vi "G#Object_GetAllObjects.vi"(1 "full class name (\"\")":string, 2 "only refs (F)":bool, 5 "error in (no error)":errorcluster) -> (10 "all objects":T1[](array[typedef]), 12 "all refs":refnum<class "G#Object.lvclass">[](array[class]), 15 "class information":T3[](array[typedef]), 19 "error out":errorcluster)   [LabVIEW 2017, in "G#Object.lvclass"]
doc: "Returns all objects of the specified class. If \"full class name\" is empty, all objects of all classes will be returned."
uses:
  G#Object.lvclass
  G#Object_ClassInfoType.ctl
  G#Object_ObjectInfoType.ctl
  G#Object_CreateMethod.ctl
  G#Object.lvclass/G#Object.ctl
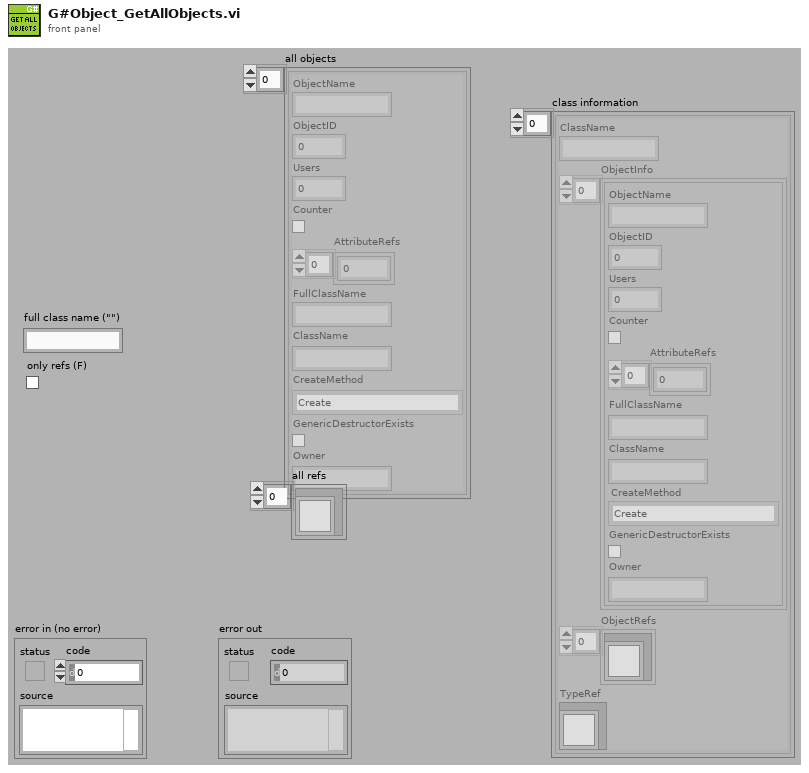
[diagram p1: front panel]
types:
  T1 = typedef "G#Object.lvclass/G#Object_ObjectInfoType.ctl" = cluster{"ObjectName":string, "ObjectID":u32, "Users":i32, "Counter":bool, "AttributeRefs":u32[], "FullClassName":string, "ClassName":string, "CreateMethod":T2, "GenericDestructorExists":bool, "Owner":string}
  T2 = typedef "G#Object.lvclass/G#Object_CreateMethod.ctl" = enum16{"Create", "Create or look up existing", "Look up existing"}
  T3 = typedef "G#Object.lvclass/G#Object_ClassInfoType.ctl" = cluster{"ClassName":string, "ObjectInfo":T1[], "ObjectRefs":refnum<class "G#Object.lvclass">[], "TypeRef":refnum<class "G#Object.lvclass">}
  T4 = cluster{"full class name (\"\")":string, "Ref":refnum<class "G#Object.lvclass">}
  T5 = cluster{"full class name (\"\")":string, "Ref":refnum<class "G#Object.lvclass">}[]
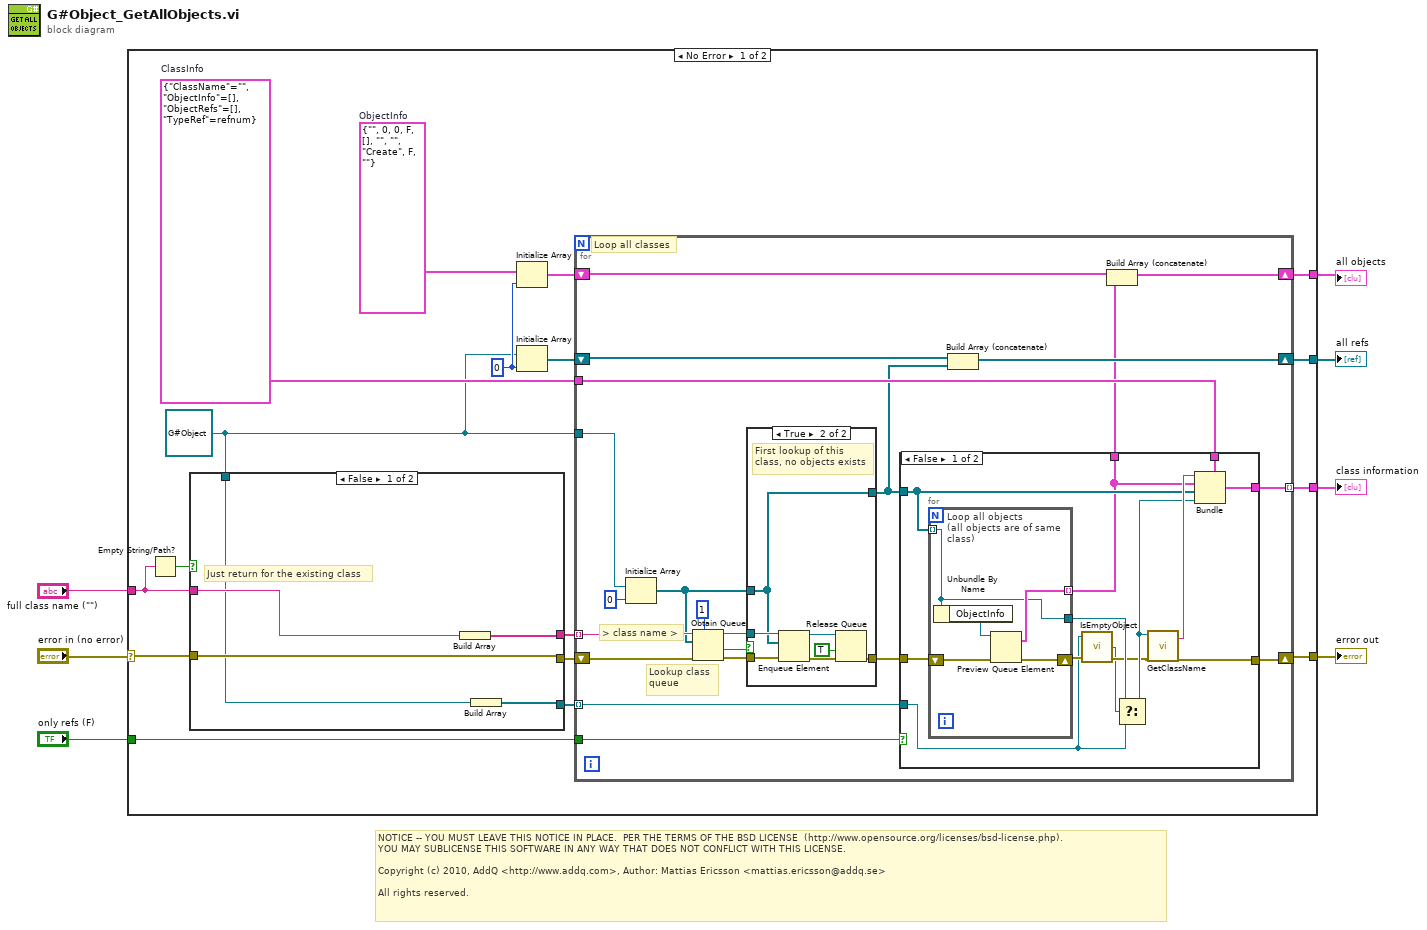
[diagram p0: block diagram]
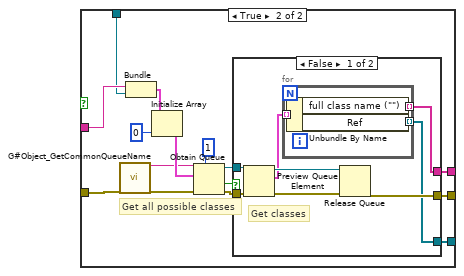
[diagram p2: hidden frame]
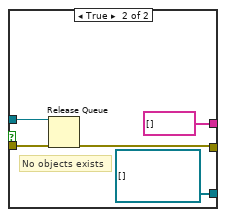
[diagram p3: hidden frame]
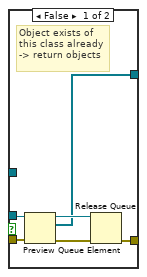
[diagram p5: hidden frame]
diagram:
  # "NOTICE -- YOU MUST LEAVE THIS NOTICE IN PLACE.  PER THE TERMS OF THE BSD LICENSE  (http://www.opensource.org/licenses/bsd-license.php).\nYOU MAY SUBLICENSE THIS SOFTWARE IN ANY WAY THAT DOES NOT CONFLICT WITH THIS LICENSE.\n\nCopyright (c) 2010, AddQ <http://www.addq.com>, Author: Mattias Ericsson <mattias.ericsson@addq.se>\n\nAll rights reserved."
  n1 = case shown="No Error" "error in (no error)" {
    selector: "error in (no error)" -> [w20 w114]
    tunnel: [w14 w114] -> w6
    tunnel: [w18 _] -> w5
    tunnel: [w19 _] -> w4
    tunnel: [w15 _] -> w3
    tunnel: "only refs (F)" -> [w13 _]
    tunnel: "full class name (\"\")" -> [w11 _]
    frame No Error {
      w9 = refnum<class "G#Object.lvclass"> refnum ("Ref")
      w10 = T1 {"ObjectName"="", "ObjectID"=0, "Users"=0, "Counter"=FALSE, "AttributeRefs"=[], "FullClassName"="", "ClassName"="", "CreateMethod"=enum."Create", "GenericDestructorExists"=FALSE, "Owner"=""}  # ObjectInfo
      w21 = T3 {"ClassName"="", "ObjectInfo"=[], "ObjectRefs"=[], "TypeRef"=refnum}  # ClassInfo
      w16 = 0 ("dimension size")
      n2 = Empty String/Path?(string/path=w11) -> (empty?=w12:bool)
      n3 = case shown="False" w12 {
        tunnel: [w28 w38] -> w23
        tunnel: [w29 w37] -> w22
        tunnel: w20 -> [w29 w32]
        tunnel: w11 -> [w27 w35]
        tunnel: w9 -> [w26 w33]
        tunnel: [w25 w34] -> w8
        frame False {
          # "Just return for the existing class"
          n4 = Build Array(w27) -> (w28:string[])
          n5 = Build Array(w26) -> (w25:refnum<class "G#Object.lvclass">[])
        }
        frame True {
          # "Get all possible classes"
          n6 = call "G#Object_GetCommonQueueName.vi"("error in (no error)"=w32) -> ("queue name"=w30:string, "error out"=w31:errorcluster)  [unwired: 17 in]
          n7 = Bundle("full class name (\"\")"=w35, "Ref"=w33) -> (w36:T4)  [unwired: 1 in]
          n8 = Initialize Array(w36, 0 ("dimension size")) -> (w39:T5)
          n9 = Obtain Queue(max queue size (-1, unlimited)=1, name (unnamed)=w30, element data type=w39, error in (no error)=w31) -> (queue out=w42:refnum<queue>, created new?=w44:bool, error out=w43:errorcluster)  [unwired: 1 in]
          n10 = case shown="False" w44 {
            tunnel: w43 -> [w52 w57]
            tunnel: w42 -> [w51 w58]
            tunnel: [w47 string[] []] -> w38
            tunnel: [w50 w60] -> w37
            tunnel: [w45 refnum<class "G#Object.lvclass">[] []] -> w34
            frame False {
              # "Get classes"
              n11 = Preview Queue Element(queue=w51, error in (no error)=w52) -> (queue out=w48:refnum<queue>, element=w46:T5, error out=w49:errorcluster)  [unwired: 1 in, 1 out]
              n12 = for {
                tunnel: [w55] -> w47 mode=indexing
                tunnel: w46 -> [w54] mode=indexing
                tunnel: [w53] -> w45 mode=indexing
                n13 = Unbundle By Name(w54) -> ("full class name (\"\")"=w55:string, "Ref"=w53:refnum<class "G#Object.lvclass">)
              }
              n14 = Release Queue(queue=w48, error in (no error)=w49) -> (error out=w50:errorcluster)  [unwired: 1 in, 2 out]
            }
            frame True {
              # "No objects exists"
              n15 = Release Queue(queue=w58, error in (no error)=w57) -> (error out=w60:errorcluster)  [unwired: 1 in, 2 out]
            }
          }
        }
      }
      n16 = Initialize Array(w10, w16) -> (w17:T1[])
      n17 = Initialize Array(w9, w16) -> (w24:refnum<class "G#Object.lvclass">[])
      n18 = for {
        shift-right: [w70] -> w14
        shift-left: w22 -> [w77]
        tunnel: w23 -> [w65] mode=indexing
        tunnel: [w76] -> w19 mode=indexing
        shift-right: [w75] -> w18
        shift-left: w24 -> [w74]
        tunnel: w9 -> [w64]
        tunnel: w21 -> [w73]
        shift-right: [w68] -> w15
        shift-left: w17 -> [w67]
        tunnel: w13 -> [w66]
        tunnel: w8 -> [w61] mode=indexing
        # "Loop all classes"
        # "> class name >"
        # "Lookup class\nqueue"
        n19 = Initialize Array(w64, 0 ("dimension size")) -> (w63:refnum<class "G#Object.lvclass">[])
        n20 = Obtain Queue(max queue size (-1, unlimited)=1, name (unnamed)=w65, element data type=w63, error in (no error)=w77) -> (queue out=w78:refnum<queue>, created new?=w79:bool, error out=w80:errorcluster)  [unwired: 1 in]
        n21 = case shown="True" w79 {
          tunnel: w80 -> [w105 w113]
          tunnel: w78 -> [w104 w112]
          tunnel: w63 -> [_ w111]
          tunnel: [w106 w110] -> w72
          tunnel: [w101 w111] -> w71
          frame False {
            # "Object exists of\nthis class already\n-> return objects"
            n22 = Preview Queue Element(queue=w104, error in (no error)=w105) -> (queue out=w102:refnum<queue>, element=w101:refnum<class "G#Object.lvclass">[], error out=w103:errorcluster)  [unwired: 1 in, 1 out]
            n23 = Release Queue(queue=w102, error in (no error)=w103) -> (error out=w106:errorcluster)  [unwired: 1 in, 2 out]
          }
          frame True {
            # "First lookup of this\nclass, no objects exists"
            n24 = Enqueue Element(queue=w112, element=w111, error in (no error)=w113) -> (queue out=w108:refnum<queue>, error out=w109:errorcluster)  [unwired: 1 in, 1 out]
            n25 = Release Queue(queue=w108, force destroy? (F)=TRUE, error in (no error)=w109) -> (error out=w110:errorcluster)  [unwired: 2 out]
          }
        }
        n26 = case shown="False" w66 {
          tunnel: [w94 _] -> w76
          tunnel: w73 -> [w93 _]
          tunnel: w72 -> [w92 w100]
          tunnel: w71 -> [w83 _]
          tunnel: [w91 w100] -> w70
          tunnel: [w82 _] -> w69
          tunnel: w61 -> [w85 _]
          frame False {
            n27 = for {
              shift-right: [w98] -> w87
              shift-left: w92 -> [w99]
              tunnel: w83 -> [w95] mode=indexing
              tunnel: [w96] -> w82 mode=indexing
              tunnel: [w95] -> w89
              # "Loop all objects\n(all objects are of same\nclass)"
              n28 = Unbundle By Name(w95) -> ("ObjectInfo"=w97:refnum<queue>)
              n29 = Preview Queue Element(queue=w97, error in (no error)=w99) -> (element=w96:T1, error out=w98:errorcluster)  [unwired: 1 in, 2 out]
            }
            n30 = call-dynamic "IsEmptyObject.vi"("error in (no error)"=w87, "reference in"=w85) -> ("error out"=w86:errorcluster, "is empty?"=w84:bool)  [unwired: 1 in, 1 out]
            n31 = Select(t=w89, s=w84, f=w85) -> (s? t:f=w88:refnum<class "G#Object.lvclass">)
            n32 = call-dynamic "GetClassName.vi"("reference in"=w88, "error in (no error)"=w86) -> ("class name"=w90:string, "error out"=w91:errorcluster)  [unwired: 13 in, 3 out]
            n33 = Bundle(cluster=w93, "ClassName"=w90, "ObjectInfo"=w82, "ObjectRefs"=w83, "TypeRef"=w88) -> (w94:T3)
          }
          frame True {
            # "Only refs are wanted, skip object info"
          }
        }
        n34 = Build Array (concatenate)(w74, w71) -> (w75:refnum<class "G#Object.lvclass">[])
        n35 = Build Array (concatenate)(w67, w69) -> (w68:T1[])
      }
    }
    frame Error {
    }
  }
  "error out" <- w6
  "class information" <- w4
  "all objects" <- w3
  "all refs" <- w5
